vi "JSON Read.vi"   [LabVIEW 2020, in "Error Provider API.lvlib"]
uses:
  <vilib>/NI VeriStand/Error Provider API/Error Provider API.lvlib
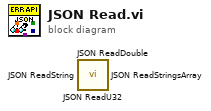
[diagram p0: block diagram]
diagram:
  n1 = call <vilib>:"JSON ReadU32.vi"() -> ()  [unwired: 10 in, 2 out]
  n2 = call <vilib>:"JSON ReadDouble.vi"() -> ()  [unwired: 10 in, 2 out]
  n3 = call <vilib>:"JSON ReadString.vi"() -> ()  [unwired: 10 in, 2 out]
  n4 = call <vilib>:"JSON ReadStringsArray.vi"() -> ()  [unwired: 10 in, 2 out]
